vi "kvCanGetVersion.vi"(0 "error in (no error)":errorcluster) -> (1 "CANLib Version (hex)":u16 format="%.0x", 2 "error out":errorcluster)   [LabVIEW 2022 SP3]
doc: "This function returns the library version number."
uses:
  canlib32.dll
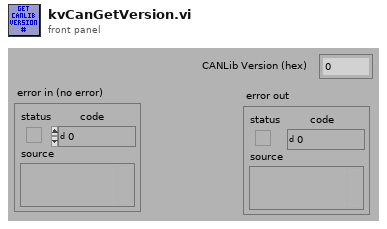
[diagram p1: front panel]
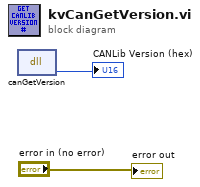
[diagram p0: block diagram]
diagram:
  n1 = dll-call lib="canlib32.dll" fn="canGetVersion"() -> (→"CANLib Version (hex)":u16)  [unwired: 3 in, 2 out]
  "error out" <- "error in (no error)"
